vi "Aspect Ratio Score.vi"(8 "Equivalent Rect Short":dbl, 9 "Equivalent Rect Long":dbl, 10 "Height":dbl, 11 "Width":dbl) -> (2 "Outer":dbl, 3 "Middle":dbl)   [LabVIEW 2012]
doc: "Compare the ratio of the rectangle to that of the expected target. Score is in percent.\n\nSince inputs are particle measurements, the diagram doesn't expect to receive zero or negative values for either input."
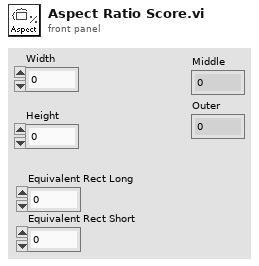
[diagram p1: front panel]
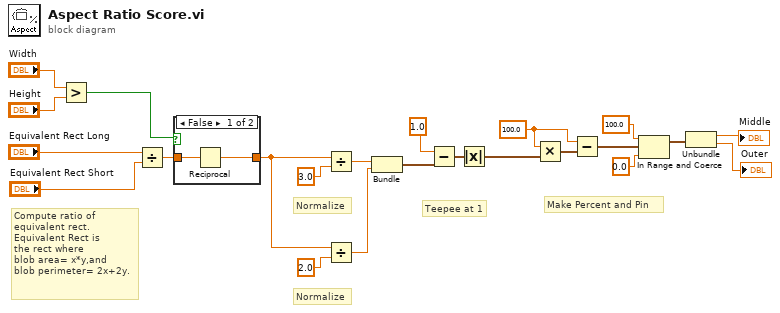
[diagram p0: block diagram]
diagram:
  w17 = 100.0 ("x/y")
  # "Make Percent and Pin"
  # "Teepee at 1"
  # "Normalize"
  # "Normalize"
  # "Compute ratio of\nequivalent rect.\nEquivalent Rect is\nthe rect where\nblob area= x*y,and\nblob perimeter= 2x+2y."
  n1 = Greater?(x="Width", y="Height") -> (0:w1:bool)
  n2 = Divide(x="Equivalent Rect Long", y="Equivalent Rect Short") -> (x/y=w3:dbl)
  n3 = case shown="False" w1 {
    tunnel: w3 -> [w25 w26]
    tunnel: [w24 w26] -> w2
    frame False {
      n4 = Reciprocal(x=w25) -> (1/x=w24:dbl)
    }
    frame True {
    }
  }
  n5 = Divide(x=w2, y=3.0) -> (x/y=w11:dbl)
  n6 = Divide(x=w2, y=2.0) -> (x/y=w10:dbl)
  n7 = Bundle(w11, w10) -> (w9:cluster{dbl, dbl})  [unwired: 1 in]
  n8 = Subtract(x=1.0 ("y"), y=w9) -> (x-y=w15:cluster{dbl, dbl})
  n9 = Absolute Value(x=w15) -> (abs(x)=w18:cluster{dbl, dbl})
  n10 = Multiply(x=w17, y=w18) -> (x*y=w19:cluster{dbl, dbl})
  n11 = Subtract(x=w17, y=w19) -> (x-y=w14:cluster{dbl, dbl})
  n12 = In Range and Coerce(upper limit=100.0, x=w14, lower limit=0.0) -> (coerced(x)=w8:cluster{dbl, dbl})  [unwired: 1 out]
  n13 = Unbundle(w8) -> (→"Middle":dbl, →"Outer":dbl)
